vi "WaveFormDataGenerator.vi"(8 "error in":errorcluster, 9 "sampling info":cluster{"Fs":dbl, "#s":dbl}={"Fs"=1000.0, "#s"=100.0}, 10 "Signal Types/Classes":T1(array[ring])=[enum."Sine Wave", enum."Square Wave", enum."Triangle Wave"], 11 "Number of Waveforms per Signal Type":i32=2500) -> (0 "error out":errorcluster, 2 "Proparties":sgl[][](array[numeric]), 3 "Generated Waveform":sgl[][](array[numeric]))   [LabVIEW 2020]
uses:
  <vilib>/numeric/Random Number (Range) DBL.vi
  <vilib>/measure/NI_MABase.lvlib
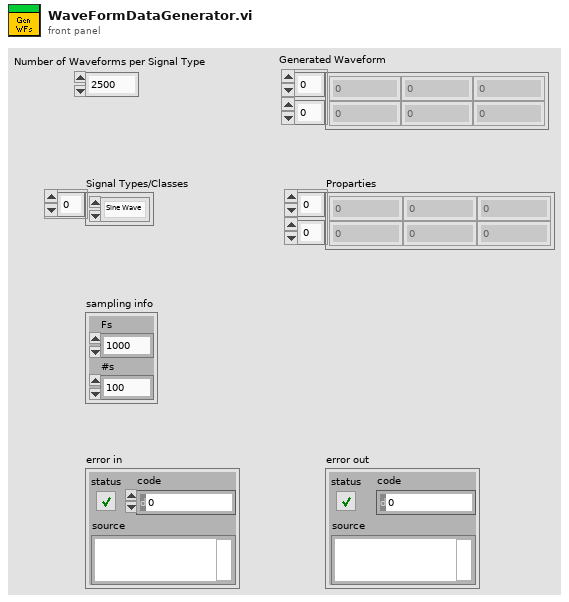
[diagram p1: front panel]
types:
  T1 = enum16{"Sine Wave", "Triangle Wave", "Square Wave", "Sawtooth Wave", "Noise"}[]
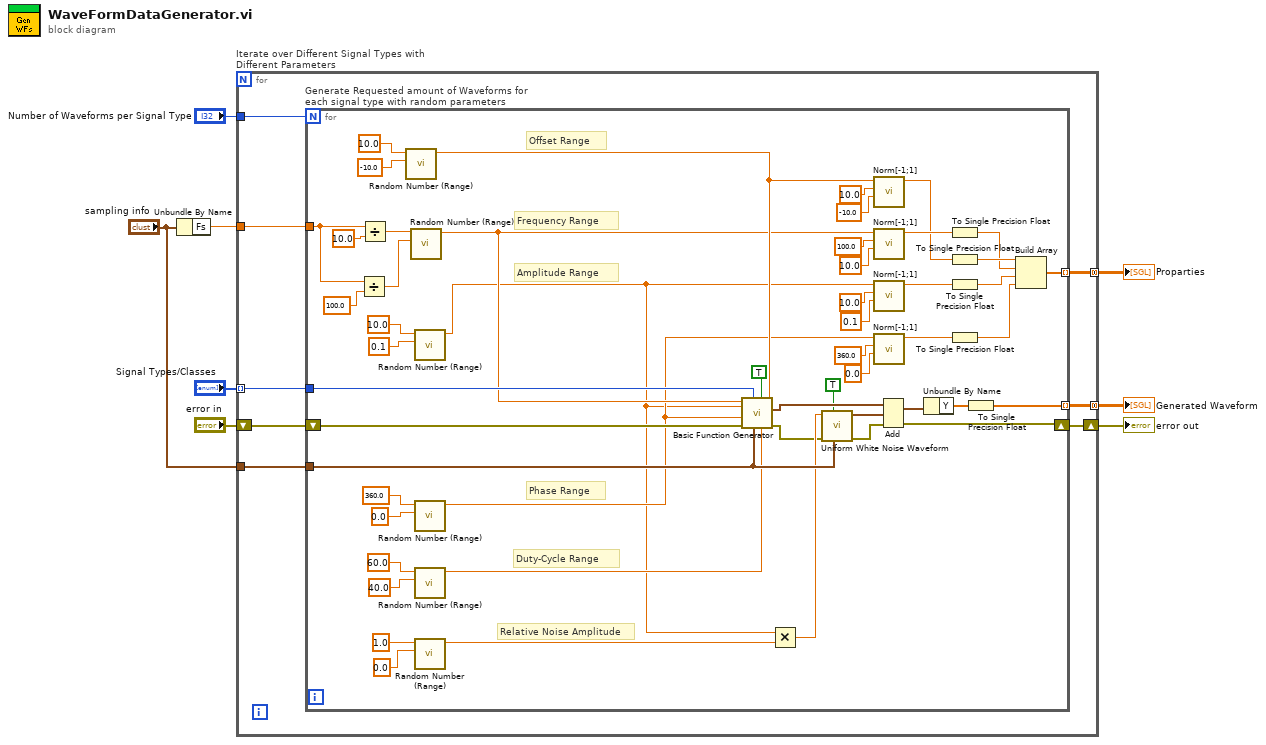
[diagram p0: block diagram]
diagram:
  n1 = Unbundle By Name("sampling info") -> ("Fs"=w8:dbl)
  n2 = for "Iterate over Different Signal Types with Different Parameters" {
    tunnel: w8 -> [w9]
    tunnel: "Number of Waveforms per Signal Type" -> [w10]
    tunnel: "sampling info" -> [w16]
    tunnel: [w13] -> w2 mode=concatenating
    tunnel: "Signal Types/Classes" -> [w12] mode=indexing
    shift-right: [w15] -> w5
    shift-left: "error in" -> [w14]
    tunnel: [w11] -> w1 mode=concatenating
    n3 = for "Generate Requested amount of Waveforms for each signal type with random parameters" {
      N: w10 -> [_]
      tunnel: [w38] -> w13 mode=indexing
      shift-right: [w67] -> w15
      shift-left: w14 -> [w68]
      tunnel: w9 -> [w62]
      tunnel: w12 -> [w64]
      tunnel: w16 -> [w51]
      tunnel: [w41] -> w11 mode=indexing
      # "Relative Noise Amplitude"
      # "Offset Range"
      # "Duty-Cycle Range"
      # "Phase Range"
      # "Amplitude Range"
      # "Frequency Range"
      n4 = Divide(x=w62, y=100.0) -> (x/y=w61:dbl)
      n5 = Divide(x=w62, y=10.0) -> (x/y=w63:dbl)
      n6 = call-poly <vilib>:"Random Number (Range).vi"("lower bound (0)"=-10.0, "upper bound (100)"=10.0) -> ("number"=w24:dbl)  [unwired: 9 in]
      n7 = call-poly <vilib>:"Random Number (Range).vi"("lower bound (0)"=w61, "upper bound (100)"=w63) -> ("number"=w23:dbl)  [unwired: 9 in]
      n8 = call-poly <vilib>:"Random Number (Range).vi"("lower bound (0)"=0.1, "upper bound (100)"=10.0) -> ("number"=w19:dbl)  [unwired: 9 in]
      n9 = call-poly <vilib>:"Random Number (Range).vi"("lower bound (0)"=0.0, "upper bound (100)"=360.0) -> ("number"=w22:dbl)  [unwired: 9 in]
      n10 = call-poly <vilib>:"Random Number (Range).vi"("lower bound (0)"=40.0, "upper bound (100)"=60.0) -> ("number"=w20:dbl)  [unwired: 9 in]
      n11 = call-poly <vilib>:"Random Number (Range).vi"("lower bound (0)"=0.0, "upper bound (100)"=1.0) -> ("number"=w21:dbl)  [unwired: 9 in]
      n12 = call <vilib>:"Basic Function Generator.vi"("offset"=w24, "square wave duty cycle (%)"=w20, "reset signal"=TRUE, "sampling info"=w51, "signal type"=w64, "error in (no error)"=w68, "phase"=w22, "amplitude"=w19, "frequency"=w23) -> ("error out"=w43:errorcluster, "signal out"=w47:waveform(dbl))  [unwired: 1 out]
      n13 = Multiply(x=w19, y=w21) -> (x*y=w45:dbl)
      n14 = call <vilib>:"Uniform White Noise Waveform.vi"("sampling info"=w51, "reset signal"=TRUE, "error in (no error)"=w43, "amplitude"=w45) -> ("error out"=w42:errorcluster, "signal out"=w44:waveform(dbl))  [unwired: 6 in]
      n15 = call "Norm[-1;1].vi"("Min"=-10.0, "Max"=10.0, "Original Value"=w24) -> ("Norm Value"=w31:dbl)  [unwired: 8 in]
      n16 = call "Norm[-1;1].vi"("Min"=10.0, "Max"=100.0, "Original Value"=w23) -> ("Norm Value"=w35:dbl)  [unwired: 8 in]
      n17 = call "Norm[-1;1].vi"("Min"=0.1, "Max"=10.0, "Original Value"=w19) -> ("Norm Value"=w28:dbl)  [unwired: 8 in]
      n18 = call "Norm[-1;1].vi"("Min"=0.0, "Max"=360.0, "Original Value"=w22) -> ("Norm Value"=w25:dbl)  [unwired: 8 in]
      n19 = Add(1:w44, 2:w47, 4:w42) -> (0:w50:waveform(dbl), 3:w67:errorcluster)
      n20 = Unbundle By Name(w50) -> ("Y"=w65:dbl[])
      n21 = To Single Precision Float(number=w35) -> (single precision float=w17:sgl)
      n22 = To Single Precision Float(number=w31) -> (single precision float=w18:sgl)
      n23 = To Single Precision Float(number=w28) -> (single precision float=w39:sgl)
      n24 = To Single Precision Float(number=w25) -> (single precision float=w37:sgl)
      n25 = To Single Precision Float(number=w65) -> (single precision float=w38:sgl[])
      n26 = Build Array(w18, w17, w39, w37) -> (w41:sgl[])
    }
  }
  "Generated Waveform" <- w2
  "error out" <- w5
  "Proparties" <- w1
